vi "EcrireLireValeurParDefaut_HoloTrackPy_link.vi"(7 "Lecture/Ecriture":enum32{"Lecture", "Ecriture"}(radio), 8 "error in (no error)":errorcluster, 11 "DefValueLinkIN":T1) -> (0 "error out":errorcluster, 1 "OK?":bool, 2 "XML File Path(duplicate)":path, 3 "DefValueLinkOUT":T1)   [LabVIEW 2025]
uses:
  defValuesLink.ctl
  <vilib>/Utility/xml.llb/Write to XML File(string).vi
  <vilib>/Utility/xml.llb/Read From XML File(string).vi
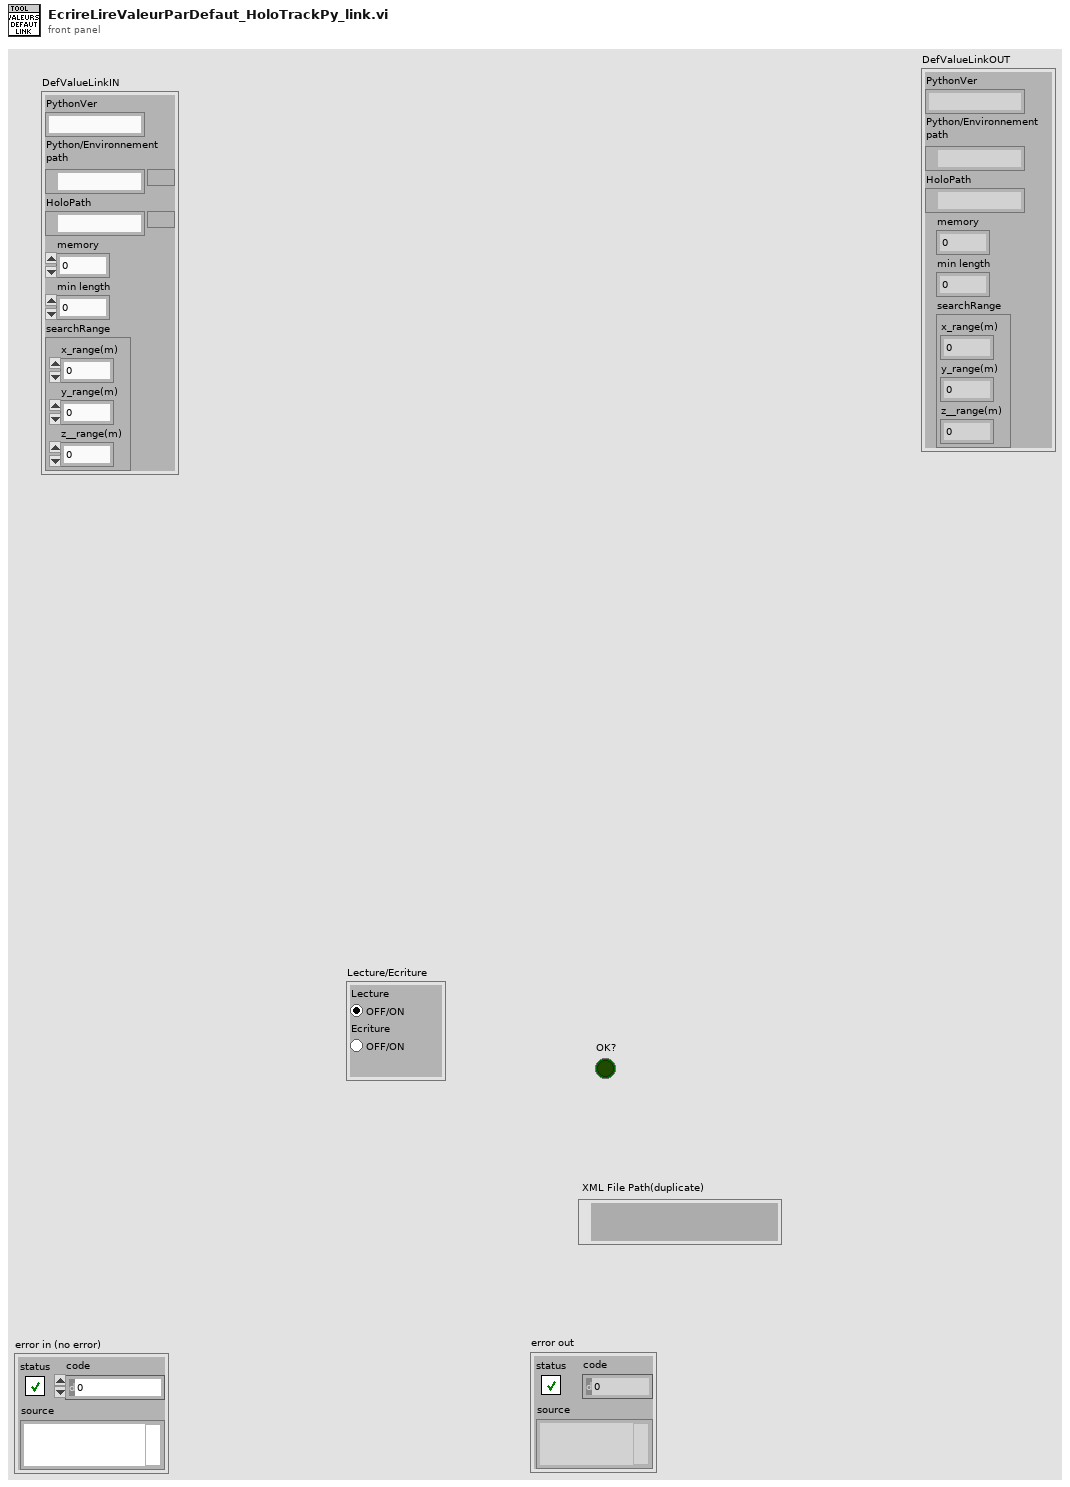
[diagram p1: front panel]
types:
  T1 = typedef "defValuesLink.ctl" = cluster{"PythonVer":string, "Python/Environnement\npath":path, "HoloPath":path, "memory":i32, "min length":i32, "searchRange":cluster{"x_range(m)":dbl, "y_range(m)":dbl, "z__range(m)":dbl}}
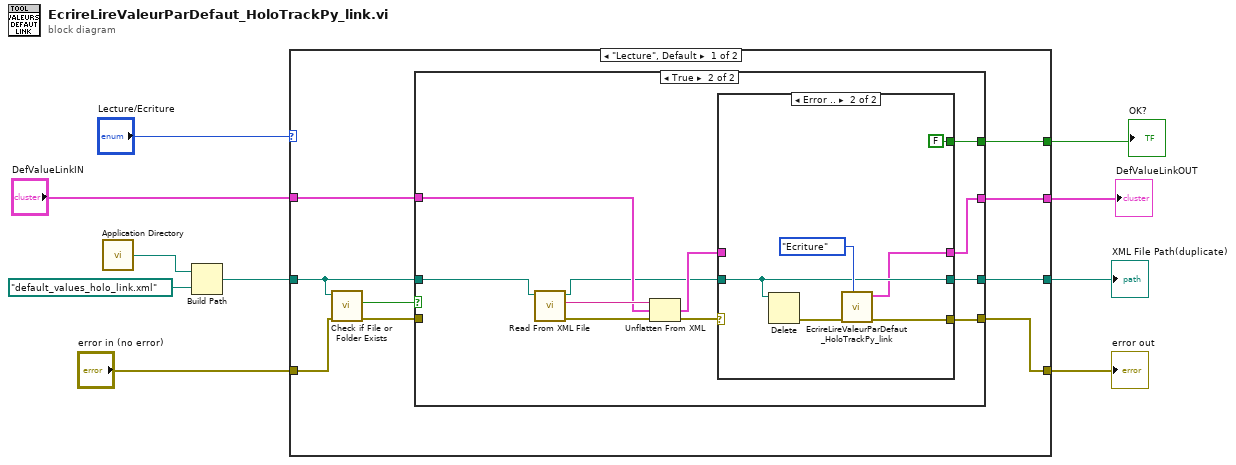
[diagram p0: block diagram]
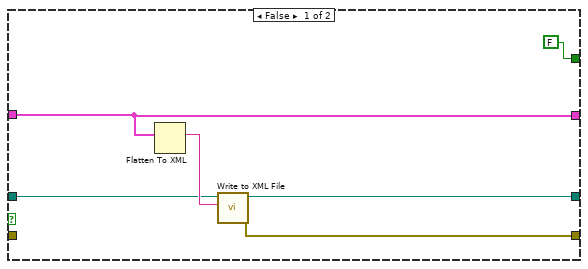
[diagram p2: hidden frame]
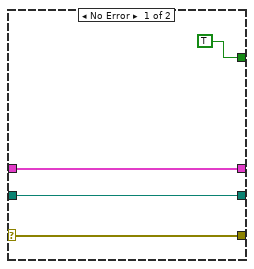
[diagram p3: hidden frame]
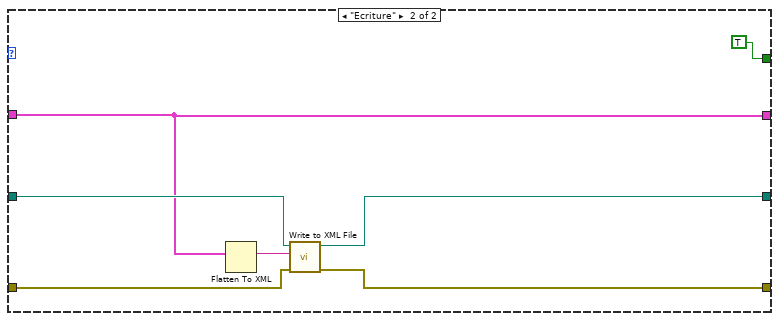
[diagram p4: hidden frame]
diagram:
  n1 = call <vilib>:"Application Directory.vi"() -> ("Application Directory"=w4:path)
  n2 = Build Path(base path=w4, name or relative path=path "default_values_holo_link.xml" ("default name")) -> (appended path=w9:path)
  n3 = case shown="\"Lecture\", Default" "Lecture/Ecriture" {
    tunnel: w9 -> [w17 w52]
    tunnel: "error in (no error)" -> [w16 w51]
    tunnel: [w18 w50] -> w7
    tunnel: [w19 w49] -> w6
    tunnel: "DefValueLinkIN" -> [w13 w48]
    tunnel: [w12 w48] -> w2
    tunnel: [w11 TRUE ("OK?")] -> w3
    frame "Lecture", Default {
      n4 = call <vilib>:"Check if File or Folder Exists.vi"("error in (no error)"=w16, "path"=w17) -> ("error out"=w15:errorcluster, "file or folder exists?"=w14:bool)  [unwired: 7 in, 1 out]
      n5 = case shown="True" w14 {
        tunnel: [w21 w30] -> w12
        tunnel: [w22 w27] -> w19
        tunnel: [w24 w31] -> w18
        tunnel: w17 -> [w23 w34]
        tunnel: w15 -> [_ _]
        tunnel: w13 -> [w21 w33]
        tunnel: [FALSE ("OK?") w26] -> w11
        frame False {
          n6 = Flatten To XML(6:w21) -> (2:w25:string)
          n7 = call-poly <vilib>:"Write to XML File.vi"("XML Input"=w25, "XML File Path"=w23) -> ("error out"=w24:errorcluster, "XML File Path(duplicate)"=w22:path)  [unwired: 3 in, 5 out]
        }
        frame True {
          n8 = call-poly <vilib>:"Read From XML File.vi"("XML File Path"=w34) -> ("error out"=w36:errorcluster, "XML Elements"=w35:string, "XML File Path(duplicate)"=w28:path)  [unwired: 8 in]
          n9 = Unflatten From XML(xml string=w35, type=w33, error in (no error)=w36) -> (value=w29:T1, error out=w32:errorcluster)
          n10 = case shown="Error .." w32 {
            selector: w32 -> [w40 _]
            tunnel: [w40 w44] -> w31
            tunnel: [w39 w41] -> w30
            tunnel: w29 -> [w39 _]
            tunnel: w28 -> [w38 w43]
            tunnel: [w38 w43] -> w27
            tunnel: [TRUE ("OK?") FALSE ("OK?")] -> w26
            frame No Error {
            }
            frame Error {
              n11 = Delete(path (use dialog)=w43) -> (error out=w46:errorcluster)  [unwired: 4 in, 2 out]
              n12 = call "EcrireLireValeurParDefaut_HoloTrackPy_link.vi"("Lecture/Ecriture"=enum32{"Lecture", "Ecriture"}."Ecriture", "error in (no error)"=w46) -> ("error out"=w44:errorcluster, "DefValueLinkOUT"=w41:T1)  [unwired: 6 in, 2 out]
            }
          }
        }
      }
    }
    frame "Ecriture" {
      n13 = Flatten To XML(6:w48) -> (2:w53:string)
      n14 = call-poly <vilib>:"Write to XML File.vi"("error in (no error)"=w51, "XML Input"=w53, "XML File Path"=w52) -> ("error out"=w50:errorcluster, "XML File Path(duplicate)"=w49:path)  [unwired: 2 in, 5 out]
    }
  }
  "error out" <- w7
  "XML File Path(duplicate)" <- w6
  "OK?" <- w3
  "DefValueLinkOUT" <- w2
